vi "扭矩动态优化.vi"(7 "SENSOR":T1, 8 "error in (no error)":errorcluster caption="错误输入（无错误）", 11 "动优化态前":cluster{dbl[], dbl[]}[](graph)) -> (0 "error out":errorcluster caption="错误输出")   [LabVIEW 2020]
uses:
  Global_Variable/Global.vi
  <userlib>/_MGI/1D Array/MGI Average/MGI Average (DBL[]).vi
panel:
  out "T2ROC1+T2ROC2+T2ROC3":i32
  out "T1ROC1+T1ROC2+T1ROC3":i32
  out "T2ROC_3":i32
  out "T1ROC_3":i32
  out "T2_AV(%)":dbl
  out "T1_AV(%)":dbl
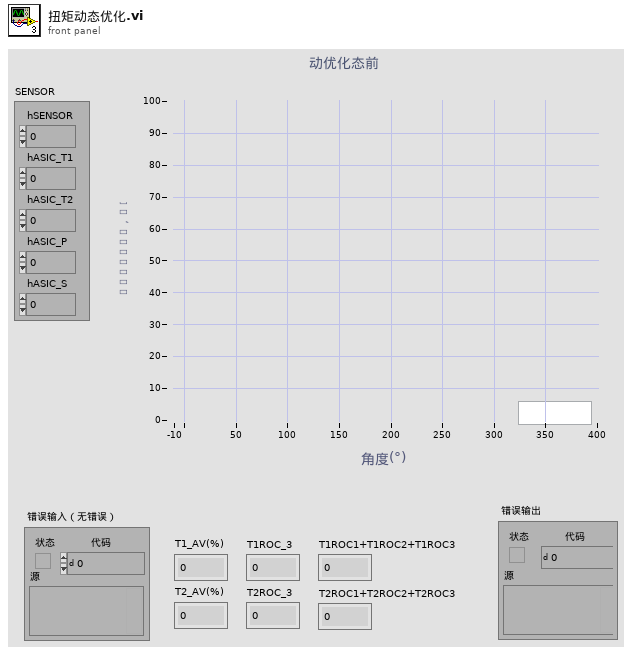
[diagram p1: front panel]
types:
  T1 = cluster{"hSENSOR":i32, "hASIC_T1":i32, "hASIC_T2":i32, "hASIC_P":i32, "hASIC_S":i32}
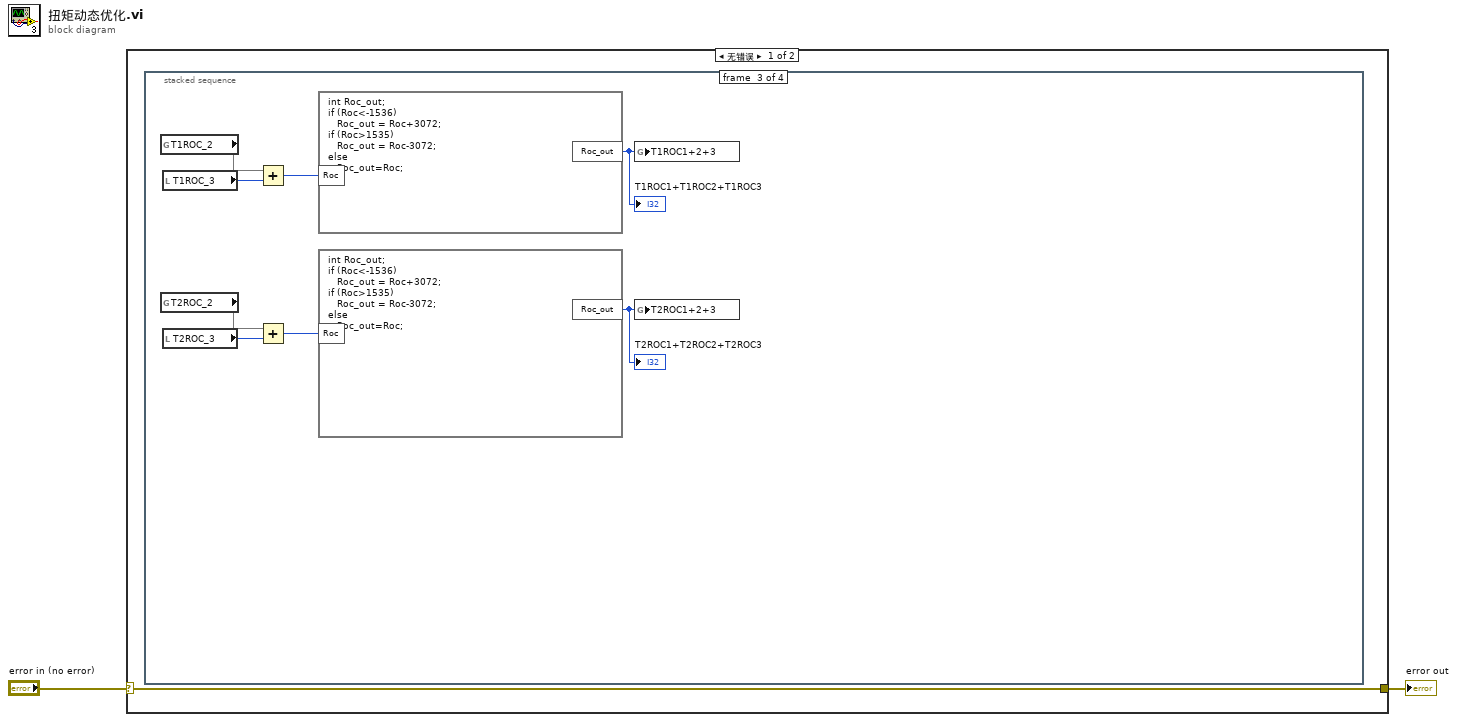
[diagram p0: block diagram]
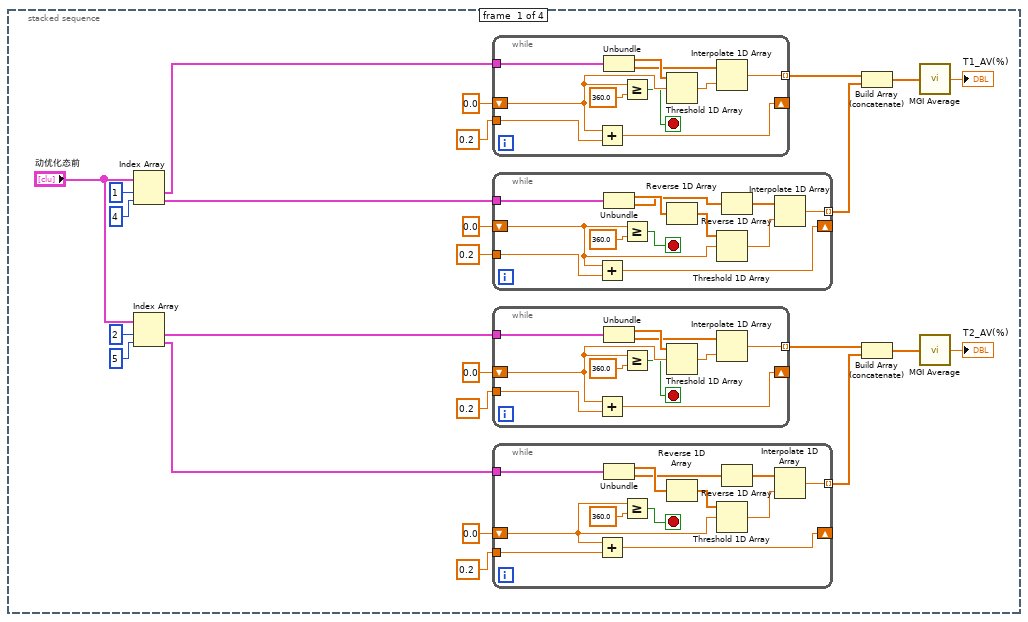
[diagram p2: hidden frame]
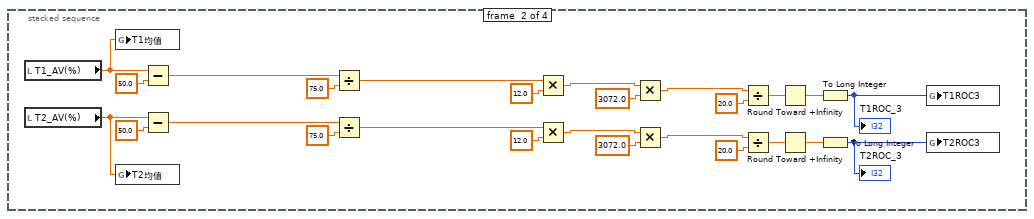
[diagram p3: hidden frame]
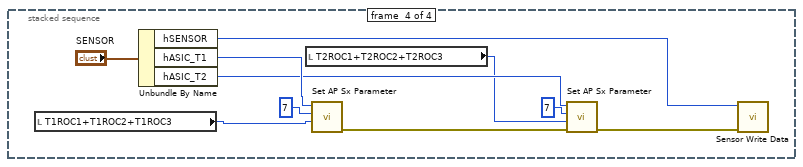
[diagram p4: hidden frame]
diagram:
  n1 = case shown="无错误" "error in (no error)" {
    selector: "error in (no error)" -> [w3 w117]
    tunnel: [w3 w117] -> w1
    frame No Error {
      n2 = stacked-sequence {
        frame #0 {
          n3 = Index Array(array="动优化态前", index #1=1 ("索引"), index #2=4 ("索引")) -> (element #1=w24:cluster{dbl[], dbl[]}, element #2=w19:cluster{dbl[], dbl[]})
          n4 = Index Array(array="动优化态前", index #1=2 ("索引"), index #2=5 ("索引")) -> (element #1=w14:cluster{dbl[], dbl[]}, element #2=w13:cluster{dbl[], dbl[]})
          n5 = while {
            tunnel: w24 -> [w72]
            shift-right: [w66] -> _
            shift-left: 0.0 -> [w65]
            tunnel: [w68] -> w12 mode=indexing
            tunnel: 0.2 -> [w67]
            stop <- w63 stop-if-true
            n6 = Add(x=w65, y=w67) -> (x+y=w66:dbl)
            n7 = Unbundle(w72) -> (w71:dbl[], w69:dbl[])
            n8 = Greater Or Equal?(x=w65, y=360.0) -> (x >= y?=w63:bool)
            n9 = Threshold 1D Array(2:w65, 3:w71) -> (0:w70:dbl)  [unwired: 1 in]
            n10 = Interpolate 1D Array(1:w70, 2:w69) -> (0:w68:dbl)
          }
          n11 = while {
            tunnel: w19 -> [w62]
            shift-right: [w56] -> _
            shift-left: 0.0 -> [w55]
            tunnel: [w58] -> w11 mode=indexing
            tunnel: 0.2 -> [w57]
            stop <- w51 stop-if-true
            n12 = Add(x=w55, y=w57) -> (x+y=w56:dbl)
            n13 = Unbundle(w62) -> (w61:dbl[], w59:dbl[])
            n14 = Greater Or Equal?(x=w55, y=360.0) -> (x >= y?=w51:bool)
            n15 = Reverse 1D Array(array=w61) -> (reversed array=w53:dbl[])
            n16 = Threshold 1D Array(2:w55, 3:w53) -> (0:w60:dbl)  [unwired: 1 in]
            n17 = Reverse 1D Array(array=w59) -> (reversed array=w52:dbl[])
            n18 = Interpolate 1D Array(1:w60, 2:w52) -> (0:w58:dbl)
          }
          n19 = while {
            tunnel: w14 -> [w50]
            shift-right: [w44] -> _
            shift-left: 0.0 -> [w43]
            tunnel: [w46] -> w7 mode=indexing
            tunnel: 0.2 -> [w45]
            stop <- w41 stop-if-true
            n20 = Add(x=w43, y=w45) -> (x+y=w44:dbl)
            n21 = Unbundle(w50) -> (w49:dbl[], w47:dbl[])
            n22 = Greater Or Equal?(x=w43, y=360.0) -> (x >= y?=w41:bool)
            n23 = Threshold 1D Array(2:w43, 3:w49) -> (0:w48:dbl)  [unwired: 1 in]
            n24 = Interpolate 1D Array(1:w48, 2:w47) -> (0:w46:dbl)
          }
          n25 = while {
            tunnel: w13 -> [w40]
            shift-right: [w34] -> _
            shift-left: 0.0 -> [w33]
            tunnel: [w36] -> w10 mode=indexing
            tunnel: 0.2 -> [w35]
            stop <- w29 stop-if-true
            n26 = Add(x=w33, y=w35) -> (x+y=w34:dbl)
            n27 = Unbundle(w40) -> (w39:dbl[], w37:dbl[])
            n28 = Greater Or Equal?(x=w33, y=360.0) -> (x >= y?=w29:bool)
            n29 = Reverse 1D Array(array=w39) -> (reversed array=w30:dbl[])
            n30 = Threshold 1D Array(2:w33, 3:w30) -> (0:w38:dbl)  [unwired: 1 in]
            n31 = Reverse 1D Array(array=w37) -> (reversed array=w31:dbl[])
            n32 = Interpolate 1D Array(1:w38, 2:w31) -> (0:w36:dbl)
          }
          n33 = Build Array (concatenate)(w12, w11) -> (w9:dbl[])
          n34 = Build Array (concatenate)(w7, w10) -> (w8:dbl[])
          n35 = call-poly <userlib>:"MGI Average.vi"("Double[]"=w9) -> ("Average"=→"T1_AV(%)":dbl)  [unwired: 1 in]
          n36 = call-poly <userlib>:"MGI Average.vi"("Double[]"=w8) -> ("Average"=→"T2_AV(%)":dbl)  [unwired: 1 in]
        }
        frame #1 {
          n37 = local read "T1_AV(%)"() -> (w74:dbl)
          n38 = local read "T2_AV(%)"() -> (w73:dbl)
          n39 = global write "Global.vi" "T1均值"(w74) -> ()
          n40 = global write "Global.vi" "T2均值"(w73) -> ()
          n41 = Subtract(x=w74, y=50.0) -> (x-y=w97:dbl)
          n42 = Subtract(x=w73, y=50.0) -> (x-y=w86:dbl)
          n43 = Divide(x=w97, y=75.0) -> (x/y=w95:dbl)
          n44 = Divide(x=w86, y=75.0) -> (x/y=w88:dbl)
          n45 = Multiply(x=w95, y=12.0) -> (x*y=w82:dbl)
          n46 = Multiply(x=w88, y=12.0) -> (x*y=w83:dbl)
          n47 = Multiply(x=w82, y=3072.0) -> (x*y=w80:dbl)
          n48 = Multiply(x=w83, y=3072.0) -> (x*y=w81:dbl)
          n49 = Divide(x=w80, y=20.0) -> (x/y=w84:dbl)
          n50 = Divide(x=w81, y=20.0) -> (x/y=w79:dbl)
          n51 = Round Toward +Infinity(x=w84) -> (ceil(x): smallest int >= x=w77:dbl)
          n52 = Round Toward +Infinity(x=w79) -> (ceil(x): smallest int >= x=w78:dbl)
          n53 = To Long Integer(number=w77) -> (32bit integer=w76:i32)
          "T1ROC_3" <- w76
          n54 = To Long Integer(number=w78) -> (32bit integer=w75:i32)
          "T2ROC_3" <- w75
          n55 = global write "Global.vi" "T1ROC3"(w76) -> ()
          n56 = global write "Global.vi" "T2ROC3"(w75) -> ()
        }
        frame #2 {
          n57 = global read "Global.vi" "T1ROC_2"() -> (w100)
          n58 = global read "Global.vi" "T2ROC_2"() -> (w99)
          n59 = local read "T1ROC_3"() -> (w106:i32)
          n60 = local read "T2ROC_3"() -> (w103:i32)
          n61 = Add(x=w100, y=w106) -> (x+y=w105:i32)
          n62 = Add(x=w99, y=w103) -> (x+y=w104:i32)
          n63 = formula code="int Roc_out;\nif (Roc<-1536)\n   Roc_out = Roc+3072;\nif (Roc>1535)\n   Roc_out = Roc-3072;\nelse\n   Roc_out=Roc;"("Roc"=w105) -> ("Roc_out"=w102:i32)
          "T1ROC1+T1ROC2+T1ROC3" <- w102
          n64 = formula code="int Roc_out;\nif (Roc<-1536)\n   Roc_out = Roc+3072;\nif (Roc>1535)\n   Roc_out = Roc-3072;\nelse\n   Roc_out=Roc;"("Roc"=w104) -> ("Roc_out"=w101:i32)
          "T2ROC1+T2ROC2+T2ROC3" <- w101
          n65 = global write "Global.vi" "T1ROC1+2+3"(w102) -> ()
          n66 = global write "Global.vi" "T2ROC1+2+3"(w101) -> ()
        }
        frame #3 {
          n67 = local read "T1ROC1+T1ROC2+T1ROC3"() -> (w109:i32)
          n68 = Unbundle By Name("SENSOR") -> ("hSENSOR"=w114:i32, "hASIC_T1"=w116:i32, "hASIC_T2"=w115:i32)
          n69 = local read "T2ROC1+T2ROC2+T2ROC3"() -> (w108:i32)
          n70 = call "Set AP Sx Parameter.vi"("para2"=w109, "asicBitsName"=7, "asicHandle"=w116) -> ("error out"=w111:errorcluster)  [unwired: 7 in, 1 out]
          n71 = call "Set AP Sx Parameter.vi"("error in (no error)"=w111, "para2"=w108, "asicBitsName"=7, "asicHandle"=w115) -> ("error out"=w110:errorcluster)  [unwired: 6 in, 1 out]
          n72 = call "Sensor Write Data.vi"("error in (no error)"=w110, "sensorHandle"=w114) -> ()  [unwired: 8 in, 2 out]
        }
      }
    }
    frame Error {
    }
  }
  "error out" <- w1
